vi "WriteText.vi"(6 "Text Color":T7=4914962, 8 "error in (no error)":errorcluster, 9 "Offset":cluster{"x":i16, "y":i16}, 11 "Data in":T1={"Class"={"Ants"=refnum, "Layer"=refnum, "Templates"=refnum, "Icon"=refnum, "Glyph"=refnum, "Settings"=refnum, "Tools"=refnum}, "Ref"={"Add Layer"=refnum, "Remove Layer"=refnum, "Line Text"=[], "Body Text Spec"=refnum, "DNL_Font"=refnum, "glyph path str"=refnum, "templates path str"=refnum, "Arrow Up"=refnum, "Arrow Down"=refnum, "IE VI Ref"=refnum, "Glyphs tree"=refnum, "Templates tree"=refnum, "Layer Icon Text"=refnum, "Layer Template"=refnum, "Clipboard"=refnum, "BW icon in"=refnum, "Color icon in"=refnum, "Layer Clust"=refnum, "Body Text"=refnum, "DNL_Framework Templates"=refnum, "Search Templates"=refnum, "TextMarker"=refnum, "Tab Control"=refnum, "Search Glyphs"=refnum, "Line Color"=refnum, "DNL_Glyphs []"=refnum, "Fill Color"=refnum, "Tools"=refnum, "Glyphs tree"=refnum, "Icon"=refnum, "Preview"=refnum, "Ants"=refnum, "Terminals"=refnum, "menu reference"=refnum, "LayerNames"=[], "GlyphLoadAnimation"=refnum, "TemplateLoadAnimation"=refnum, "refreshGlyphs"=refnum, "refreshTemplates"=refnum}, "Support"={"AntsRect"={"left"=0, "top"=0, "right"=0, "bottom"=0}, "Mouse Move Coords"={"Horizontal"=0, "Vertical"=0}, "Mouse Down Coords"={"Horizontal"=0, "Vertical"=0}, "Temp Coord"={"Horizontal"=0, "Vertical"=0}, "Action"=enum."Default", "Edge Color"=4914962, "Fill Color"=16860, "Mouse Down?"=FALSE, "Draft Mode?"=FALSE, "Temp Icon"=bytes[3102], "CTRL Pressed"=FALSE, "Move Selection?"=FALSE, "AntsRect Orig"={"left"=0, "top"=0, "right"=0, "bottom"=0}, "Text"="", "TM Set?"=FALSE, "Mouse inside icon?"=FALSE, "Tool (old value)"=0, "Pencil Move Color"=0, "Swap Colors?"=FALSE, "Shift pressed?"=FALSE}}) -> (0 "error out":errorcluster, 2 "Picture":picture, 3 "Data out":T1={"Class"={"Ants"=refnum, "Layer"=refnum, "Templates"=refnum, "Icon"=refnum, "Glyph"=refnum, "Settings"=refnum, "Tools"=refnum}, "Ref"={"Add Layer"=refnum, "Remove Layer"=refnum, "Line Text"=[], "Body Text Spec"=refnum, "DNL_Font"=refnum, "glyph path str"=refnum, "templates path str"=refnum, "Arrow Up"=refnum, "Arrow Down"=refnum, "IE VI Ref"=refnum, "Glyphs tree"=refnum, "Templates tree"=refnum, "Layer Icon Text"=refnum, "Layer Template"=refnum, "Clipboard"=refnum, "BW icon in"=refnum, "Color icon in"=refnum, "Layer Clust"=refnum, "Body Text"=refnum, "DNL_Framework Templates"=refnum, "Search Templates"=refnum, "TextMarker"=refnum, "Tab Control"=refnum, "Search Glyphs"=refnum, "Line Color"=refnum, "DNL_Glyphs []"=refnum, "Fill Color"=refnum, "Tools"=refnum, "Glyphs tree"=refnum, "Icon"=refnum, "Preview"=refnum, "Ants"=refnum, "Terminals"=refnum, "menu reference"=refnum, "LayerNames"=[], "GlyphLoadAnimation"=refnum, "TemplateLoadAnimation"=refnum, "refreshGlyphs"=refnum, "refreshTemplates"=refnum}, "Support"={"AntsRect"={"left"=0, "top"=0, "right"=0, "bottom"=0}, "Mouse Move Coords"={"Horizontal"=0, "Vertical"=0}, "Mouse Down Coords"={"Horizontal"=0, "Vertical"=0}, "Temp Coord"={"Horizontal"=0, "Vertical"=0}, "Action"=enum."Default", "Edge Color"=4914962, "Fill Color"=16860, "Mouse Down?"=FALSE, "Draft Mode?"=FALSE, "Temp Icon"=bytes[3102], "CTRL Pressed"=FALSE, "Move Selection?"=FALSE, "AntsRect Orig"={"left"=0, "top"=0, "right"=0, "bottom"=0}, "Text"="", "TM Set?"=FALSE, "Mouse inside icon?"=FALSE, "Tool (old value)"=0, "Pencil Move Color"=0, "Swap Colors?"=FALSE, "Shift pressed?"=FALSE}})   [LabVIEW 2021]
uses:
  <vilib>/LabVIEW Icon API/lv_icon/Controls/IEColor.ctl
  <resource>/plugins/NIIconEditor/Controls/IE Data.ctl
  <resource>/plugins/NIIconEditor/Class/Ants/Ants.lvclass
  <resource>/plugins/NIIconEditor/Class/FakedArray/FakedArray.lvclass
  <resource>/plugins/NIIconEditor/Class/Icon Library/Glyph.lvclass
  <resource>/plugins/NIIconEditor/Class/Settings/Settings.lvclass
  <resource>/plugins/NIIconEditor/Class/Tools/Tools Paint.lvclass
  <vilib>/LabVIEW Icon API/lv_icon/Classes/Icon/Icon.lvclass
  <resource>/plugins/NIIconEditor/Controls/IE Classes.ctl
  <resource>/plugins/NIIconEditor/Controls/References Cluster.ctl
  <resource>/plugins/NIIconEditor/Controls/SupportClass.ctl
  <vilib>/Utility/miscctls.llb/LVPoint32TypeDef.ctl
  <resource>/plugins/NIIconEditor/Controls/SupportClass_Action.ctl
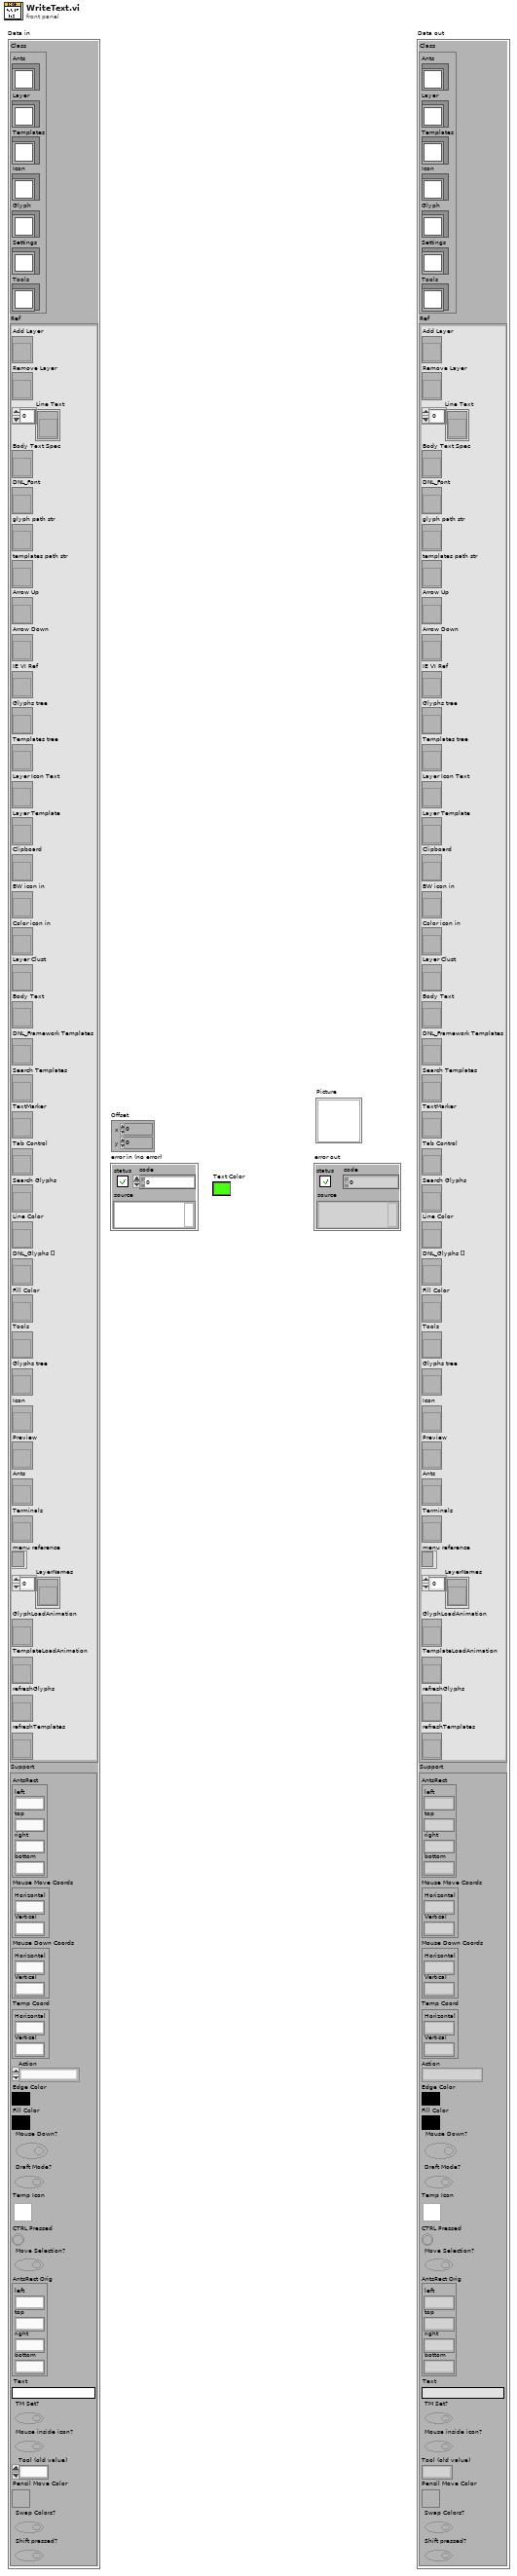
[diagram p1: front panel]
types:
  T1 = typedef "IE Data.ctl" = cluster{"Class":T2, "Ref":T3, "Support":T4}
  T2 = typedef "IE Classes.ctl" = cluster{"Ants":refnum<class "Ants.lvclass">, "Layer":refnum<class "FakedArray.lvclass">, "Templates":refnum<class "FakedArray.lvclass">, "Icon":refnum<class "Icon.lvclass">, "Glyph":refnum<class "Glyph.lvclass">, "Settings":refnum<class "Settings.lvclass">, "Tools":refnum<class "Tools Paint.lvclass">}
  T3 = typedef "References Cluster.ctl" = cluster{"Add Layer":refnum<vi>, "Remove Layer":refnum<vi>, "Line Text":refnum<vi>[], "Body Text Spec":refnum<vi>, "DNL_Font":refnum<vi>, "glyph path str":refnum<vi>, "templates path str":refnum<vi>, "Arrow Up":refnum<vi>, "Arrow Down":refnum<vi>, "IE VI Ref":refnum<vi>, "Glyphs tree":refnum<vi>, "Templates tree":refnum<vi>, "Layer Icon Text":refnum<vi>, "Layer Template":refnum<vi>, "Clipboard":refnum<vi>, "BW icon in":refnum<vi>, "Color icon in":refnum<vi>, "Layer Clust":refnum<vi>, "Body Text":refnum<vi>, "DNL_Framework Templates":refnum<vi>, "Search Templates":refnum<vi>, "TextMarker":refnum<vi>, "Tab Control":refnum<vi>, "Search Glyphs":refnum<vi>, "Line Color":refnum<vi>, "DNL_Glyphs []":refnum<vi>, "Fill Color":refnum<vi>, "Tools":refnum<vi>, "Glyphs tree":refnum<vi>, "Icon":refnum<vi>, "Preview":refnum<vi>, "Ants":refnum<vi>, "Terminals":refnum<vi>, "menu reference":refnum<k9>, "LayerNames":refnum<vi>[], "GlyphLoadAnimation":refnum<vi>, "TemplateLoadAnimation":refnum<vi>, "refreshGlyphs":refnum<vi>, "refreshTemplates":refnum<vi>}
  T4 = typedef "SupportClass.ctl" = cluster{"AntsRect":cluster{"left":i16, "top":i16, "right":i16, "bottom":i16}, "Mouse Move Coords":T5, "Mouse Down Coords":T5, "Temp Coord":T5, "Action":T6, "Edge Color":T7, "Fill Color":T7, "Mouse Down?":bool, "Draft Mode?":bool, "Temp Icon":picture, "CTRL Pressed":bool, "Move Selection?":bool, "AntsRect Orig":cluster{"left":i16, "top":i16, "right":i16, "bottom":i16}, "Text":string, "TM Set?":bool, "Mouse inside icon?":bool, "Tool (old value)":u32, "Pencil Move Color":u32, "Swap Colors?":bool, "Shift pressed?":bool}
  T5 = typedef "LVPoint32TypeDef.ctl" = cluster{"Horizontal":i32, "Vertical":i32}
  T6 = typedef "SupportClass_Action.ctl" = enum16{"Default", "Move Selection", "Glyph Library", "Tool"}
  T7 = typedef "IEColor.ctl" = u32
  T8 = enum16{"User-specified Font", "Application Font", "System Font", "Dialog Font"}
  T9 = cluster{"Font Name:":string, "Size":i16, "Strikeout?":bool, "Italic?":bool, "Underline?":bool, "Outline?":bool, "Shadow?":bool, "Bold?":bool}
  T10 = cluster{"horizontal":enum16{"left", "center", "right"}, "vertical":enum16{"top", "center", "bottom"}}
  T11 = typedef "Font.ctl" = string
  T12 = typedef "Alignment.ctl" = u16
  T13 = typedef "Font Size.ctl" = u8
  T14 = cluster{"left":i16, "top":i16, "right":i16, "bottom":i16}
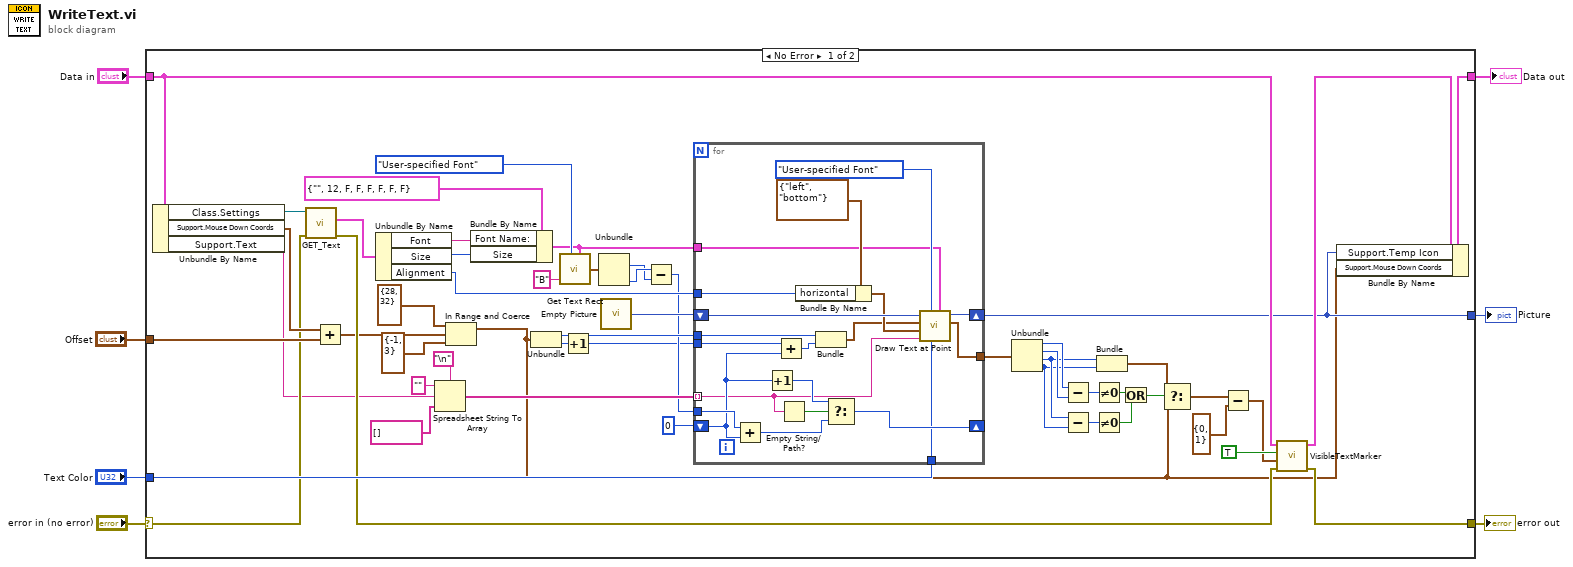
[diagram p0: block diagram]
diagram:
  n1 = case shown="No Error" "error in (no error)" {
    selector: "error in (no error)" -> [w18 w81]
    tunnel: [w37 w81] -> w6
    tunnel: [w13 _] -> w5
    tunnel: "Offset" -> [w31 _]
    tunnel: "Text Color" -> [w38 _]
    tunnel: "Data in" -> [w17 w80]
    tunnel: [w14 w80] -> w1
    frame No Error {
      n2 = Unbundle By Name(w17) -> ("Class.Settings"=w20:refnum<class "Settings.lvclass">, "Support.Mouse Down Coords"=w19:T5, "Support.Text"=w15:string)
      n3 = call-dynamic "GET_Text.vi"("error in (no error)"=w18, "Settings.lvclass in"=w20) -> ("error out"=w35:errorcluster, "Text"=w49:cluster{"Font":T11, "Alignment":T12, "Size":T13})  [unwired: 8 out]
      n4 = Add(x=w19, y=w31) -> (x+y=w11:T5)
      n5 = Unbundle By Name(w49) -> ("Font"=w51:T11, "Size"=w52:T13, "Alignment"=w48:T12)
      n6 = Spreadsheet String To Array(delimiter (Tab)="\n", format string="", spreadsheet string=w15, array type (2D Dbl)=string[] []) -> (array=w57:string[])
      n7 = In Range and Coerce(upper limit=T5 {"Horizontal"=28, "Vertical"=32}, x=w11, lower limit=T5 {"Horizontal"=-1, "Vertical"=3}) -> (coerced(x)=w10:T5)  [unwired: 1 out]
      n8 = Bundle By Name(cluster=T9 {"Font Name:"="", "Size"=12, "Strikeout?"=FALSE, "Italic?"=FALSE, "Underline?"=FALSE, "Outline?"=FALSE, "Shadow?"=FALSE, "Bold?"=FALSE} ("[user-specified font]"), "Font Name:"=w51, "Size"=w52) -> (w42:T9)
      n9 = Unbundle(w10) -> ("Horizontal"=w55:i32, "Vertical"=w54:i32)
      n10 = call <vilib>:"Get Text Rect.vi"("desired font(Application)"=T8."User-specified Font", "text"="B", "[user-specified font]"=w42) -> ("rect"=w46:T14)  [unwired: 3 in, 3 out]
      n11 = Increment(x=w54) -> (x+1=w39:i32)
      n12 = Unbundle(w46) -> ("top"=w43:i16, "bottom"=w44:i16)  [unwired: 2 out]
      n13 = call "Empty Picture"() -> ("empty picture"=w56:picture)
      n14 = Subtract(x=w44, y=w43) -> (x-y=w41:i16)
      n15 = for {
        tunnel: w57 -> [w62] mode=indexing
        shift-right: [w78] -> w13
        shift-left: w56 -> [w79]
        tunnel: w55 -> [w74]
        tunnel: w39 -> [w72]
        tunnel: w48 -> [w70]
        tunnel: w42 -> [w69]
        shift-right: [w64] -> _
        shift-left: 0 -> [w66]
        tunnel: w41 -> [w67]
        tunnel: [w61] -> w34
        tunnel: w38 -> [w60]
        n16 = Add(x=w67, y=w66) -> (x+y=w65:i32)
        n17 = Increment(x=w66) -> (x+1=w68:i32)
        n18 = Add(x=w72, y=w66) -> (x+y=w73:i32)
        n19 = Empty String/Path?(string/path=w62) -> (empty?=w63:bool)
        n20 = Bundle By Name(cluster=T10 {"horizontal"=enum."left", "vertical"=enum."bottom"} ("alignment(left, top)"), "horizontal"=w70) -> (w76:T10)
        n21 = Bundle("Horizontal"=w74, w73) -> (w71:cluster{"Horizontal":i32, i32})  [unwired: 1 out]
        n22 = Select(t=w68, s=w63, f=w65) -> (s? t:f=w64:i32)
        n23 = call <vilib>:"Draw Text at Point.vi"("[user-specified font]"=w69, "text color(black)"=w60, "desired font(Application)"=T8."User-specified Font", "text"=w62, "alignment(left, top)"=w76, "origin"=w71, "picture"=w79) -> ("text rect"=w61:T14, "new picture"=w78:picture)  [unwired: 2 in, 1 out]
      }
      n24 = Unbundle(w34) -> ("left"=w30:i16, "top"=w29:i16, "right"=w28:i16, "bottom"=w27:i16)
      n25 = Subtract(x=w30, y=w29) -> (x-y=w26:i16)
      n26 = Subtract(x=w28, y=w27) -> (x-y=w25:i16)
      n27 = Not Equal To 0?(x=w26) -> (x != 0?=w24:bool)
      n28 = Not Equal To 0?(x=w25) -> (x != 0?=w23:bool)
      n29 = Bundle("right"=w28, "bottom"=w27) -> (w33:cluster{"right":i16, "bottom":i16})  [unwired: 1 out]
      n30 = Or(x=w24, y=w23) -> (x .or. y?=w22:bool)
      n31 = Select(t=w33, s=w22, f=w10) -> (s? t:f=w32:T5)
      n32 = Subtract(x=w32, y=cluster{"right":i16, "bottom":i16} {"right"=0, "bottom"=1}) -> (x-y=w12:T5)
      n33 = call <resource>:"VisibleTextMarker.vi"("error in (no error)"=w35, "Position"=w12, "Visible"=TRUE, "Data in"=w17) -> ("error out"=w37:errorcluster, "Data out"=w16:T1)  [unwired: 6 out]
      n34 = Bundle By Name(cluster=w16, "Support.Temp Icon"=w13, "Support.Mouse Down Coords"=w10) -> (w14:T1)
    }
    frame Error {
    }
  }
  "error out" <- w6
  "Picture" <- w5
  "Data out" <- w1
